vi "CheckTags.vi"(6 "Masks":string, 9 "Wafer":string, 10 "Die":string, 11 "StatusIn":refnum<vi>) -> (3 "StatusOut":refnum<vi>)   [LabVIEW 2020]
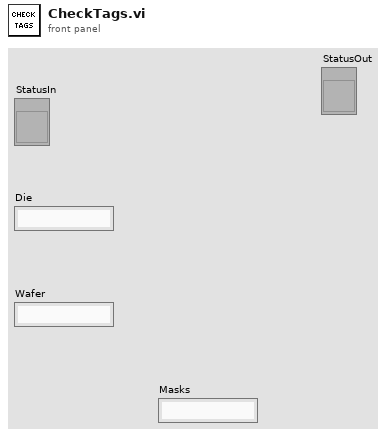
[diagram p1: front panel]
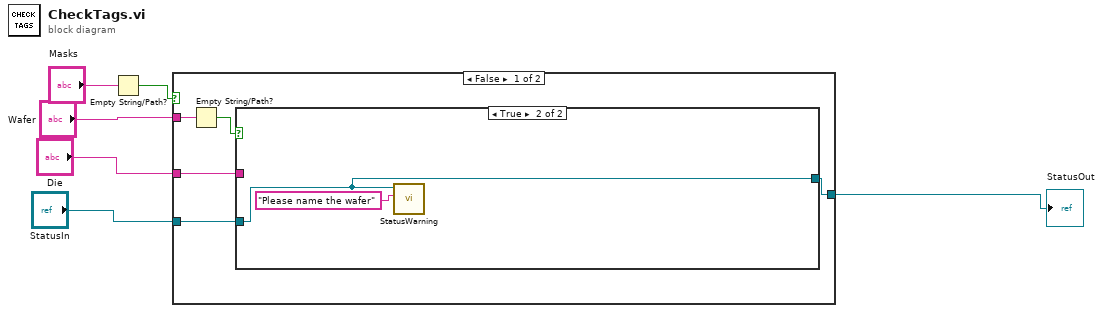
[diagram p0: block diagram]
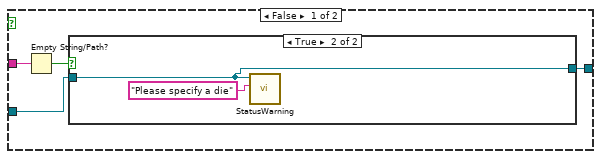
[diagram p2: hidden frame]
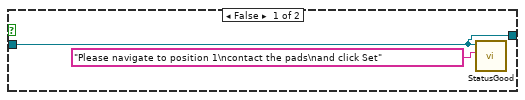
[diagram p3: hidden frame]
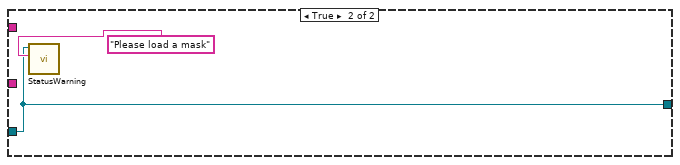
[diagram p4: hidden frame]
diagram:
  n1 = Empty String/Path?(string/path="Masks") -> (empty?=w2:bool)
  n2 = case shown="False" w2 {
    tunnel: "StatusIn" -> [w9 w22]
    tunnel: "Wafer" -> [w11 _]
    tunnel: "Die" -> [w8 _]
    tunnel: [w7 w22] -> w1
    frame False {
      n3 = Empty String/Path?(string/path=w11) -> (empty?=w10:bool)
      n4 = case shown="True" w10 {
        tunnel: w9 -> [w13 w20]
        tunnel: w8 -> [w15 _]
        tunnel: [w12 w20] -> w7
        frame False {
          n5 = Empty String/Path?(string/path=w15) -> (empty?=w14:bool)
          n6 = case shown="True" w14 {
            tunnel: w13 -> [w16 w18]
            tunnel: [w16 w18] -> w12
            frame False {
              n7 = call "StatusGood.vi"("Text.Text"="Please navigate to position 1\ncontact the pads\nand click Set", "String in"=w16) -> ()  [unwired: 10 in]
            }
            frame True {
              n8 = call "StatusWarning.vi"("Text.Text"="Please specify a die", "String in"=w18) -> ()  [unwired: 10 in]
            }
          }
        }
        frame True {
          n9 = call "StatusWarning.vi"("Text.Text"="Please name the wafer", "String in"=w20) -> ()  [unwired: 10 in]
        }
      }
    }
    frame True {
      n10 = call "StatusWarning.vi"("Text.Text"="Please load a mask", "String in"=w22) -> ()  [unwired: 10 in]
    }
  }
  "StatusOut" <- w1
